vi "Read Frequency.vi"(8 "error in (no error)":errorcluster, 11 "PWM in":refnum<class "LINX-PCA9865 PWM.lvclass">) -> (0 "error out":errorcluster, 2 "Frequency (Hz)":dbl, 3 "PWM out":refnum<class "LINX-PCA9865 PWM.lvclass">)   [LabVIEW 2019, in "LINX-PCA9865 PWM.lvclass"]
uses:
  LINX-PCA9865 PWM.lvclass
panel:
  out "Prescaler (raw)":u8
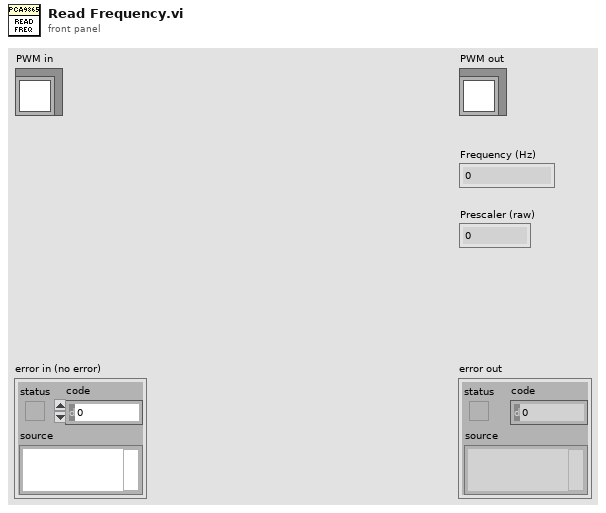
[diagram p1: front panel]
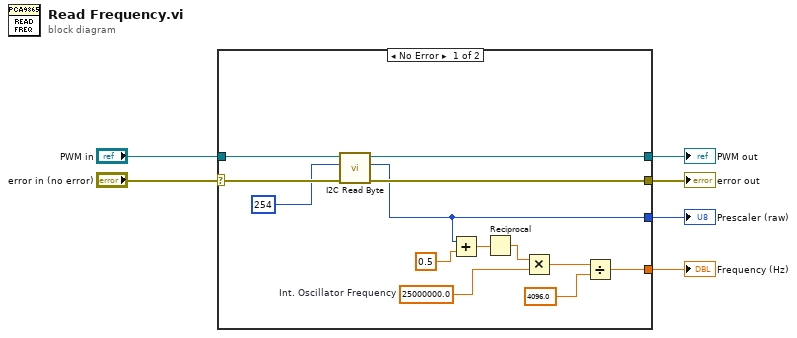
[diagram p0: block diagram]
diagram:
  n1 = case shown="No Error" "error in (no error)" {
    selector: "error in (no error)" -> [w18 w21]
    tunnel: [w16 w21] -> w5
    tunnel: [w17 w20] -> w3
    tunnel: "PWM in" -> [w19 w20]
    tunnel: [w12 _] -> w2
    tunnel: [w8 _] -> w1
    frame No Error {
      w11 = 25000000.0  # Int. Oscillator Frequency
      n2 = call "I2C Read Byte.vi"("error in (no error)"=w18, "Address"=u8 254 ("I2C Slave Address 2"), "LINX-PCA9865 PWM in"=w19) -> ("error out"=w16:errorcluster, "Byte Read"=w8:u8, "LINX-PCA9865 PWM out"=w17:refnum<class "LINX-PCA9865 PWM.lvclass">)  [unwired: 6 in]
      n3 = Add(x=w8, y=0.5 ("x")) -> (x+y=w10:dbl)
      n4 = Reciprocal(x=w10) -> (1/x=w9:dbl)
      n5 = Multiply(x=w9, y=w11) -> (x*y=w14:dbl)
      n6 = Divide(x=w14, y=4096.0 ("x")) -> (x/y=w12:dbl)
    }
    frame Error {
    }
  }
  "error out" <- w5
  "PWM out" <- w3
  "Frequency (Hz)" <- w2
  "Prescaler (raw)" <- w1
